vi "Write Skipped.vi"(11 "Assertion Result In":refnum<class "Assertion Result.lvclass">) -> (3 "Assertion Result Out":refnum<class "Assertion Result.lvclass">)   [LabVIEW 2020, in "Assertion Result.lvclass"]
uses:
  Assertion Result.lvclass
  Public/TypeDefs/Status.ctl
  Assertion Result.lvclass/Assertion Result.ctl
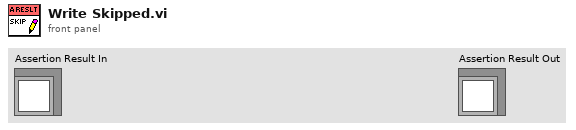
[diagram p1: front panel]
types:
  T1 = typedef "Assertion Result.lvclass/Status.ctl" = enum16{"Pass", "Fail", "Error", "Skipped", "Setup Error", "Broken", "Teardown Error"}
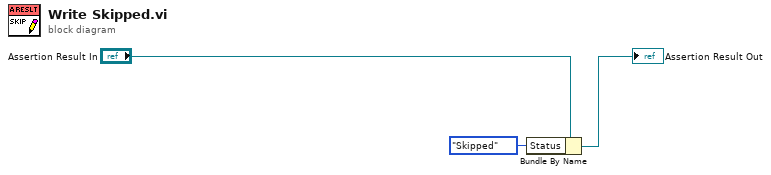
[diagram p0: block diagram]
diagram:
  n1 = Bundle By Name(cluster="Assertion Result In", "Status"=Status."Skipped") -> (→"Assertion Result Out":refnum<class "Assertion Result.lvclass">)
